vi "SP Array To Matrix - CA2.vi"(1 "Complex 2D Array":cdb[][](array[numeric])) -> (0 "Complex Matrix":T1)   [LabVIEW 2011]
doc: "Converts an array to a matrix of elements of the same type as the array elements. The data type you wire to the <B>Real 2D Array</B> input determines the polymorphic instance to use."
uses:
  TypeDefs/SP Complex Matrix.ctl
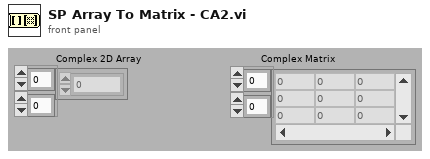
[diagram p1: front panel]
types:
  T1 = typedef "SP Complex Matrix.ctl" = cdb[][]
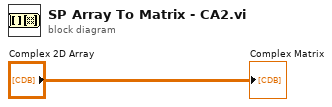
[diagram p0: block diagram]
diagram:
  "Complex Matrix" <- "Complex 2D Array"
